vi "InternalResource.vi"(7 "action":T1, 10 "count":i32, 11 "name":string) -> (2 "wait list":string[](array[string]), 3 "active list":string[](array[string]))   [LabVIEW 2017, in "McsaResourceScheduler.lvlib"]
uses:
  <vilib>/addons/InsightCM/Devices/Shared/Mcsa/McsaResourceScheduler/McsaResourceScheduler.lvlib
  <vilib>/addons/InsightCM/Devices/Shared/Mcsa/McsaResourceScheduler/controls/InternalAction.ctl
panel:
  out "error out":errorcluster
  in  "error in (no error)":errorcluster
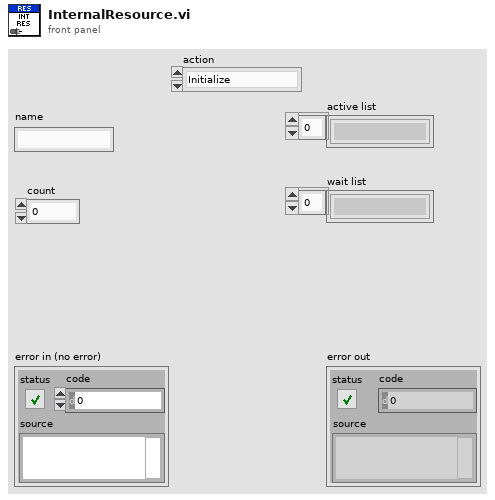
[diagram p1: front panel]
types:
  T1 = typedef "McsaResourceScheduler.lvlib/InternalAction.ctl" = enum16{"Initialize", "Register", "Unregister", "Get"}
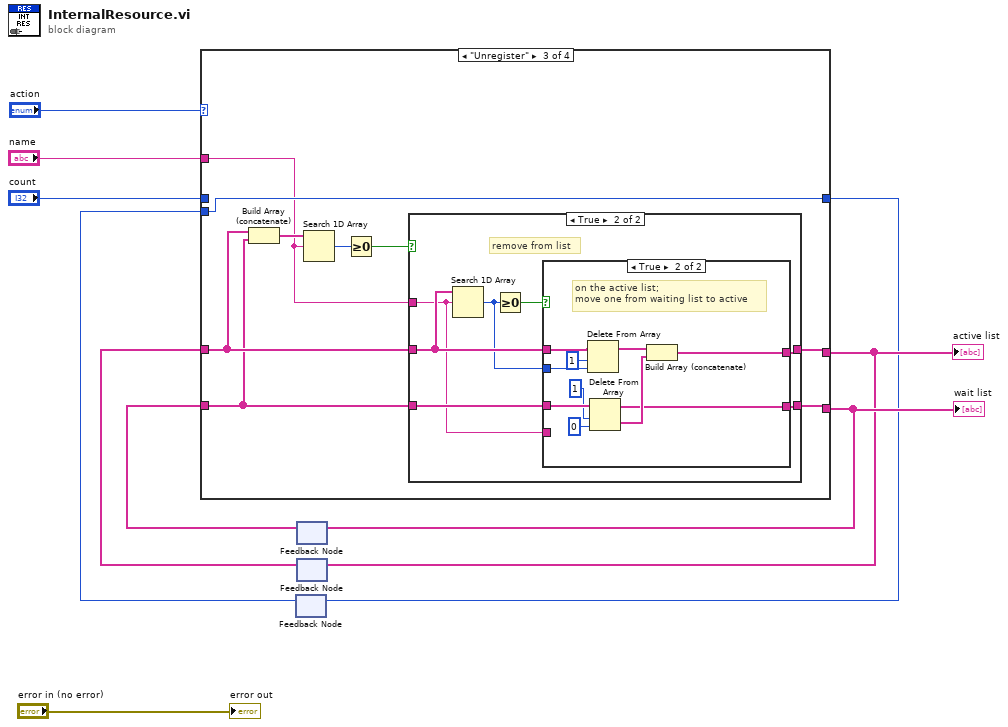
[diagram p0: block diagram]
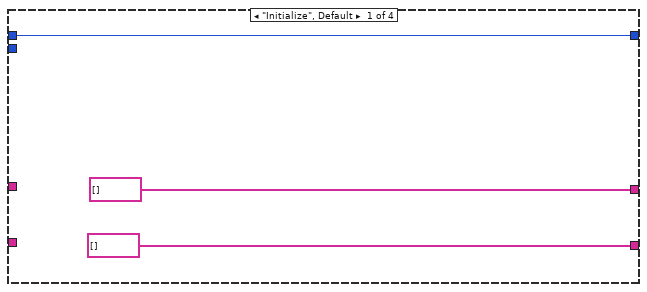
[diagram p2: hidden frame]
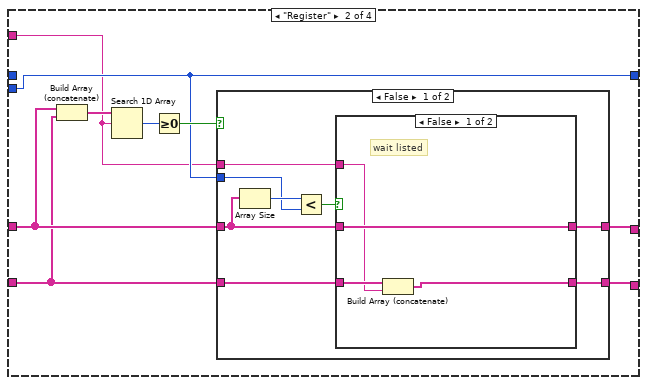
[diagram p3: hidden frame]
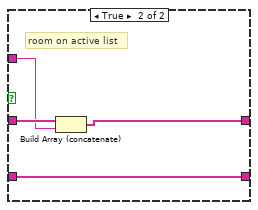
[diagram p4: hidden frame]
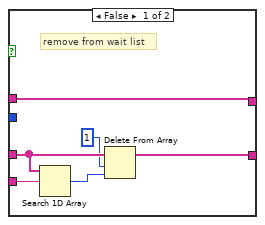
[diagram p7: hidden frame]
diagram:
  n1 = feedback #1() -> (w2:i32)  [unwired: 1 in]
  n2 = feedback #2() -> (w7:string[])  [unwired: 1 in]
  n3 = feedback #3() -> (w5:string[])  [unwired: 1 in]
  n4 = case shown="\"Unregister\"" "action" {
    tunnel: [string[] [] w18 w44 w76] -> w6
    tunnel: [string[] [] w16 w42 w75] -> w8
    tunnel: w7 -> [_ w17 w43 w75]
    tunnel: w5 -> [_ w19 w45 w76]
    tunnel: [w11 w15 w49 w77] -> w3
    tunnel: "count" -> [w11 _ _ _]
    tunnel: w2 -> [_ w15 w49 w77]
    tunnel: "name" -> [_ w14 w41 _]
    frame "Initialize", Default {
    }
    frame "Register" {
      n5 = Build Array (concatenate)(w19, w17) -> (w22:string[])
      n6 = Search 1D Array(1D array=w22, element=w14) -> (index of element=w21:i32)  [unwired: 1 in]
      n7 = Greater Or Equal To 0?(x=w21) -> (x >= 0?=w20:bool)
      n8 = case shown="False" w20 {
        tunnel: w19 -> [w27 w40]
        tunnel: [w24 w40] -> w18
        tunnel: w17 -> [w26 w39]
        tunnel: [w23 w39] -> w16
        tunnel: w15 -> [w29 _]
        tunnel: w14 -> [w25 _]
        frame False {
          n9 = Array Size(array=w27) -> (size(s)=w30:i32)
          n10 = Less?(x=w30, y=w29) -> (x < y?=w28:bool)
          n11 = case shown="False" w28 {
            tunnel: w27 -> [w34 w38]
            tunnel: w26 -> [w33 w35]
            tunnel: w25 -> [w32 w37]
            tunnel: [w34 w36] -> w24
            tunnel: [w31 w35] -> w23
            frame False {
              # "wait listed"
              n12 = Build Array (concatenate)(w33, w32) -> (w31:string[])
            }
            frame True {
              # "room on active list"
              n13 = Build Array (concatenate)(w38, w37) -> (w36:string[])
            }
          }
        }
        frame True {
          # "already registered"
        }
      }
    }
    frame "Unregister" {
      n14 = Build Array (concatenate)(w45, w43) -> (w48:string[])
      n15 = Search 1D Array(1D array=w48, element=w41) -> (index of element=w47:i32)  [unwired: 1 in]
      n16 = Greater Or Equal To 0?(x=w47) -> (x >= 0?=w46:bool)
      n17 = case shown="True" w46 {
        tunnel: w45 -> [w51 w57]
        tunnel: [w51 w54] -> w44
        tunnel: w43 -> [w50 w55]
        tunnel: [w50 w53] -> w42
        tunnel: w41 -> [_ w52]
        frame False {
          # "not registered"
        }
        frame True {
          # "remove from list"
          n18 = Search 1D Array(1D array=w57, element=w52) -> (index of element=w56:i32)  [unwired: 1 in]
          n19 = Greater Or Equal To 0?(x=w56) -> (x >= 0?=w58:bool)
          n20 = case shown="True" w58 {
            tunnel: w57 -> [w64 w74]
            tunnel: w56 -> [_ w73]
            tunnel: w55 -> [w62 w72]
            tunnel: [w64 w65] -> w54
            tunnel: [w60 w69] -> w53
            tunnel: w52 -> [w63 _]
            frame False {
              # "remove from wait list"
              n21 = Search 1D Array(1D array=w62, element=w63) -> (index of element=w61:i32)  [unwired: 1 in]
              n22 = Delete From Array(array=w62, length=1, index=w61) -> (array with subset deleted=w60:string[])  [unwired: 1 out]
            }
            frame True {
              # "on the active list;\nmove one from waiting list to active"
              n23 = Delete From Array(array=w74, length=1, index=w73) -> (array with subset deleted=w67:string[])  [unwired: 1 out]
              n24 = Delete From Array(array=w72, length=1, index=0) -> (deleted portion=w70:string[], array with subset deleted=w69:string[])
              n25 = Build Array (concatenate)(w67, w70) -> (w65:string[])
            }
          }
        }
      }
    }
    frame "Get" {
    }
  }
  "active list" <- w6
  "wait list" <- w8
  n26 = feedback-in #1(w3) -> ()
  n27 = feedback-in #2(w8) -> ()
  n28 = feedback-in #3(w6) -> ()
  "error out" <- "error in (no error)"
